vi "RampDown.vi"(1 "Output":dbl) -> (0 "Numeric":dbl)   [LabVIEW 2019]
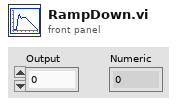
[diagram p1: front panel]
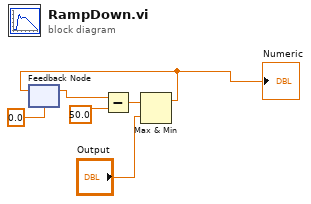
[diagram p0: block diagram]
diagram:
  n1 = feedback #1(0.0) -> (w2:dbl)
  n2 = Subtract(x=w2, y=50.0) -> (x-y=w3:dbl)
  n3 = Max & Min(x=w3, y="Output") -> (max(x,y)=w1:dbl)  [unwired: 1 out]
  "Numeric" <- w1
  n4 = feedback-in #1(w1) -> ()
